vi "Q.Swap Function RTN Q.vi"(10 "RtnQ In":refnum<queue>, 11 "Q.Element":T1) -> (2 "Exit":bool, 3 "Q.Element Out":T1)   [LabVIEW 2024, in "EQMF.lvlib" / "Queue Utils.lvlib"]
doc: "This VI enqueues a Task:\n Queue element 'Cmd' = \"Task\"\n Queue element 'Sub' is assigned to the value of the 'Task Name' input.\n\nThis VI obtains the queue by name or by queue reference.\nIf the 'Q Name' input is empty then it obtains the queue by the 'Q In\" reference.\nIf the 'Q Name' input is NOT empty then it obtains the queue by the this name.\n If a queue is ontained by name and the queue does not already exits, an error is generated.\n\nThe 'Top of Q' input is FALSE by default.\nThis input will cause this item to be enqueued on the top of the queue when it is TRUE."
uses:
  Queue Utils.lvlib
  Q.Element.ctl
  Q.Msg Return Info.ctl
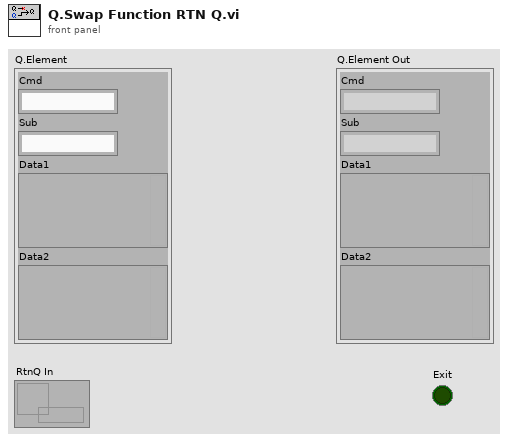
[diagram p1: front panel]
types:
  T1 = typedef "EQMF.lvlib/Queue Utils.lvlib/Q.Element.ctl" = cluster{"Cmd":string, "Sub":string, "Data1":variant, "Data2":variant}
  T2 = typedef "EQMF.lvlib/Queue Utils.lvlib/Q.Msg Return Info.ctl" = cluster{"Ret Q":refnum<queue>, "Ret Msg":T1, "SeqNum":i32}
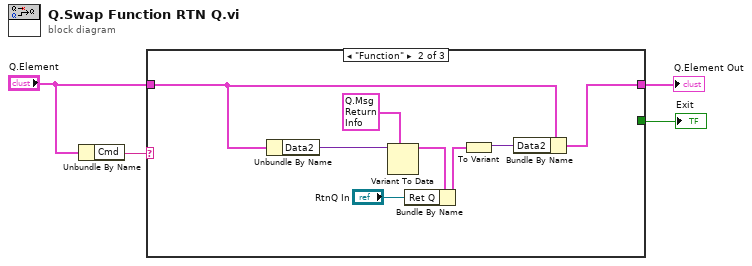
[diagram p0: block diagram]
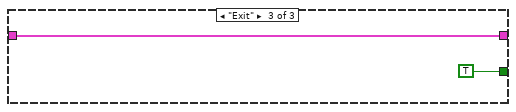
[diagram p3: hidden frame]
diagram:
  n1 = Unbundle By Name("Q.Element") -> ("Cmd"=w4:string)
  n2 = case shown="\"Function\"" w4 {
    tunnel: "Q.Element" -> [w5 w7 w14]
    tunnel: [w5 w6 w14] -> w2
    tunnel: [_ _ TRUE] -> w1
    frame Default {
    }
    frame "Function" {
      n3 = Unbundle By Name(w7) -> ("Data2"=w8:variant)
      n4 = Variant To Data(type=T2 {"Ret Q"=refnum, "Ret Msg"={"Cmd"="", "Sub"="", "Data1"=variant, "Data2"=variant}, "SeqNum"=0} ("Cmd Ret Req Data"), Variant=w8) -> (data=w10:T2)  [unwired: 1 in, 1 out]
      n5 = Bundle By Name(cluster=w10, "Ret Q"="RtnQ In") -> (w13:T2)
      n6 = To Variant(anything=w13) -> (Variant=w9:variant)
      n7 = Bundle By Name(cluster=w7, "Data2"=w9) -> (w6:T1)
    }
    frame "Exit" {
    }
  }
  "Q.Element Out" <- w2
  "Exit" <- w1
